vi "read_csv.vi"(4 "csv_file":path) -> (2 "all rows":dbl[][](array[numeric]))   [LabVIEW 2020]
uses:
  X.ctl
  Y.ctl
  <vilib>/Utility/file.llb/Read Delimited Spreadsheet (DBL).vi
panel:
  out "Y":T1
  out "X":T2
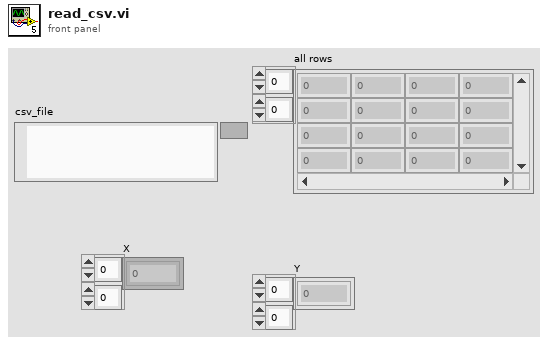
[diagram p1: front panel]
types:
  T1 = typedef "Y.ctl" = dbl[][]
  T2 = typedef "X.ctl" = dbl[][]
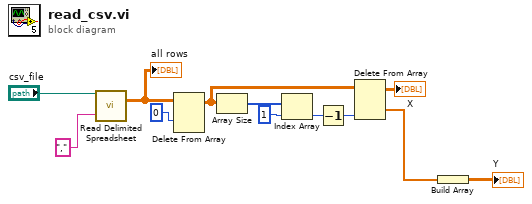
[diagram p0: block diagram]
diagram:
  n1 = call-poly <vilib>:"Read Delimited Spreadsheet.vi"("file path (dialog if empty)"="csv_file", "delimiter (\\t)"="," ("delimiter (\\t)")) -> ("all rows"=w10:dbl[][])  [unwired: 8 in, 5 out]
  "all rows" <- w10
  n2 = Delete From Array(array=w10, index (row)=0) -> (array with subset deleted=w8:dbl[][])  [unwired: 2 in, 1 out]
  n3 = Array Size(array=w8) -> (size(s)=w7:i32[])
  n4 = Index Array(array=w7, index=1) -> (element=w5:i32)
  n5 = Decrement(x=w5) -> (x-1=w4:i32)
  n6 = Delete From Array(array=w8, index (col)=w4) -> (deleted portion=w2:dbl[], array with subset deleted=→"X":dbl[][])  [unwired: 2 in]
  n7 = Build Array(w2) -> (→"Y":dbl[][])
